vi "Lvi Channel List Properties.vi"(8 "error in (no error)":errorcluster, 11 "TaskRef":i32) -> (0 "error out":errorcluster, 1 "Count":u32, 2 "CGLDepth":u32, 3 "TaskRef out":i32, 5 "function return":u32(ring))   [LabVIEW 2022 SP3, in "DtLvLink.lvlib"]
doc: "Calls directly into the entry points of the DLL of the Data Acq SDK to return information about the channel-gain list. This VI is used by the higher-level VI, DtOLGetChanList."
uses:
  DtLvLink.lvlib
  <userlib>/LV-Link3/DtLvLink_64.dll
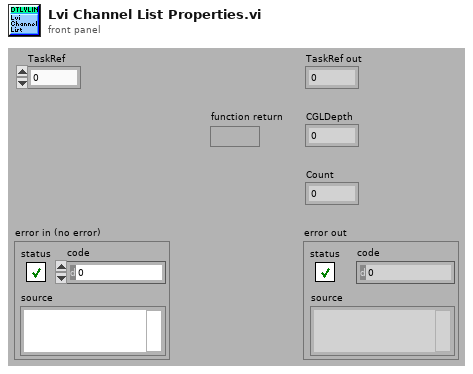
[diagram p1: front panel]
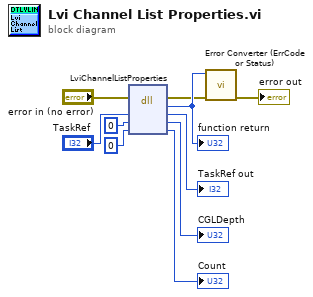
[diagram p0: block diagram]
diagram:
  n1 = dll-call lib="C:/Program Files/National Instruments/LabVIEW 2022/user.lib/LV-Link3/DtLvLink_64.*" fn="LviChannelListProperties"(error in="error in (no error)", "TaskRef"="TaskRef", "CGLDepth"=u32 0, "Count"=u32 0) -> (error out=w2:errorcluster, w10:u32, "TaskRef"=→"TaskRef out":i32, "CGLDepth"=→"CGLDepth":u32, "Count"=→"Count":u32)  [unwired: 2 in, 1 out]
  "function return" <- w10
  n2 = call "Error Converter (ErrCode or Status).vi"("error in (no error)"=w2, "error code"=w10) -> ("error out"=→"error out":errorcluster)  [unwired: 9 in]
